vi "Dispose.vi"(8 "error in (no error)":errorcluster, 11 "Actor in":refnum<class "Actor.lvclass">) -> (0 "error out":errorcluster, 3 "Actor out":refnum<class "Actor.lvclass">)   [LabVIEW 2020, in "CameraTestingProxy.lvlib" / "CameraTestingENI.lvclass"]
uses:
  CameraTestingENI.lvclass
  <vilib>/ActorFramework/Actor/Actor.lvclass
  C:/Program Files (x86)/National Instruments/LabVIEW 2020/vi.lib/ActorFramework/Actor/Actor.lvclass
  CameraTestingENI.lvclass/CameraTestingENI.ctl
  E:/GitHub/Evaluation_Test/Labview/src/CameraTestingProxy/CameraTestingENI/CameraTestingENI.lvclass
  E:/GitHub/Evaluation_Test/Labview/src/CameraTestingApp/ICameraTestingUI/ICameraTestingUI/ICameraTestingUI.lvclass
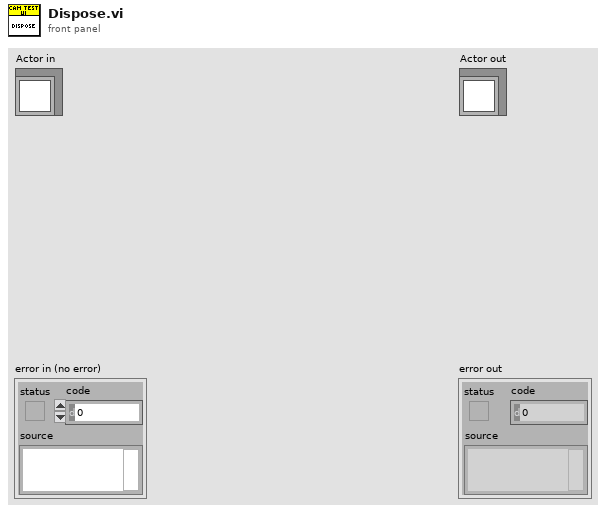
[diagram p1: front panel]
types:
  T1 = typedef "CameraTestingProxy.lvlib/CameraTestingENI.lvclass/QuitActorEvn.ctl" = refnum<user-event>
  T2 = typedef "CameraTestingProxy.lvlib/CameraTestingENI.lvclass/HelperLoopEvntRegRef.ctl" = refnum<event-registration>
  T3 = typedef "CameraTestingProxy.lvlib/CameraTestingENI.lvclass/VideoLoopEnvRgstRef.ctl" = refnum<event-registration>
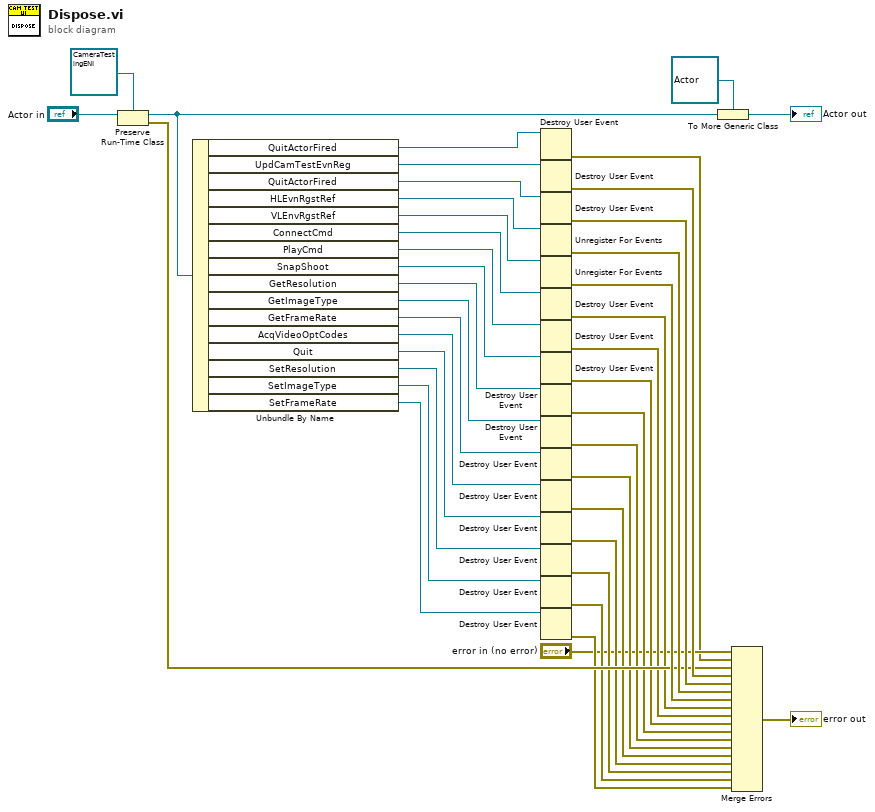
[diagram p0: block diagram]
diagram:
  n1 = Preserve Run-Time Class(object in="Actor in", 2:refnum<class "CameraTestingENI.lvclass"> refnum ("CameraTestingUI.lvlib:CameraTestingUI.lvclass")) -> (object out=w34:refnum<class "CameraTestingENI.lvclass">, error out=w26:errorcluster)  [unwired: 1 in]
  n2 = Unbundle By Name(w34) -> ("QuitActorFired"=w3:T1, "UpdCamTestEvnReg"=w40:refnum<user-event>, "QuitActorFired"=w39:T1, "HLEvnRgstRef"=w38:T2, "VLEnvRgstRef"=w37:T3, "ConnectCmd"=w25:refnum<user-event>, "PlayCmd"=w24:refnum<user-event>, "SnapShoot"=w23:refnum<user-event>, "GetResolution"=w22:refnum<user-event>, "GetImageType"=w21:refnum<user-event>, "GetFrameRate"=w20:refnum<user-event>, "AcqVideoOptCodes"=w19:refnum<user-event>, "Quit"=w18:refnum<user-event>, "SetResolution"=w17:refnum<user-event>, "SetImageType"=w16:refnum<user-event>, "SetFrameRate"=w15:refnum<user-event>)
  n3 = Destroy User Event(user event=w3) -> (error out=w1:errorcluster)  [unwired: 1 in]
  n4 = Destroy User Event(user event=w40) -> (error out=w27:errorcluster)  [unwired: 1 in]
  n5 = Destroy User Event(user event=w39) -> (error out=w28:errorcluster)  [unwired: 1 in]
  n6 = Unregister For Events(event registration refnum=w38) -> (error out=w29:errorcluster)  [unwired: 1 in]
  n7 = Unregister For Events(event registration refnum=w37) -> (error out=w30:errorcluster)  [unwired: 1 in]
  n8 = Destroy User Event(user event=w25) -> (error out=w14:errorcluster)  [unwired: 1 in]
  n9 = Destroy User Event(user event=w24) -> (error out=w13:errorcluster)  [unwired: 1 in]
  n10 = Destroy User Event(user event=w23) -> (error out=w12:errorcluster)  [unwired: 1 in]
  n11 = Destroy User Event(user event=w22) -> (error out=w11:errorcluster)  [unwired: 1 in]
  n12 = Destroy User Event(user event=w21) -> (error out=w10:errorcluster)  [unwired: 1 in]
  n13 = Destroy User Event(user event=w20) -> (error out=w9:errorcluster)  [unwired: 1 in]
  n14 = Destroy User Event(user event=w19) -> (error out=w8:errorcluster)  [unwired: 1 in]
  n15 = Destroy User Event(user event=w18) -> (error out=w7:errorcluster)  [unwired: 1 in]
  n16 = Destroy User Event(user event=w17) -> (error out=w6:errorcluster)  [unwired: 1 in]
  n17 = Destroy User Event(user event=w16) -> (error out=w5:errorcluster)  [unwired: 1 in]
  n18 = Destroy User Event(user event=w15) -> (error out=w4:errorcluster)  [unwired: 1 in]
  n19 = To More Generic Class(target class=refnum<class "Actor.lvclass"> refnum ("Actor in"), reference=w34) -> (generic class reference=→"Actor out":refnum<class "Actor.lvclass">)
  n20 = Merge Errors("error in (no error)", w1, w26, w27, w28, w29, w30, w14, w13, w12, w11, w10, w9, w8, w7, w6, w5, w4) -> (→"error out":errorcluster)
